vi "OAT Find Time Indices.vi"(7 "reset? (True)":bool=TRUE, 9 "time range":cluster{"start":dbl, "end":dbl, "step":dbl} {"step" format="%.2f"; "end" format="%.2f"; "start" format="%.2f"}, 10 "pulse/revolution (1)":i32=1, 11 "speed profile":T1 {"speed [RPM]" format="%.2f"; "time [s]" format="%.2f"}) -> (0 "finished":bool, 1 "time scale":cluster{"offset":dbl, "multiplier":dbl} {"multiplier" format="%.2f"; "offset" format="%.2f"}, 3 "rev indices":dbl[](array[numeric]) format="%.2f", 5 "last revolution":dbl format="%.2f")   [LabVIEW 2017]
uses:
  <vilib>/addons/Sound and Vibration/Order Analysis/Tach Process/SubVIs/speed profile.ctl
  <vilib>/addons/Sound and Vibration/Order Analysis/Tach Process/SoundVib_TachProcess.lvlib
panel:
  out "missing":bool
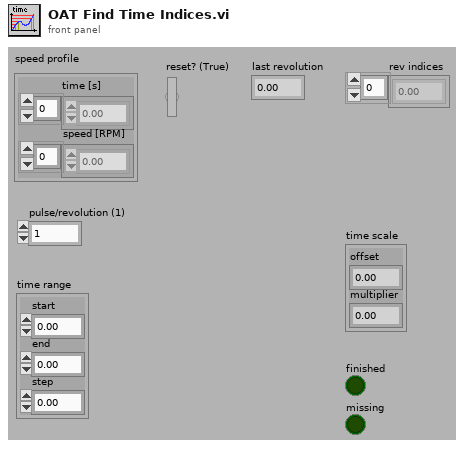
[diagram p1: front panel]
types:
  T1 = typedef "SoundVib_TachProcess.lvlib/speed profile.ctl" = cluster{"time [s]":dbl[], "speed [RPM]":dbl[]}
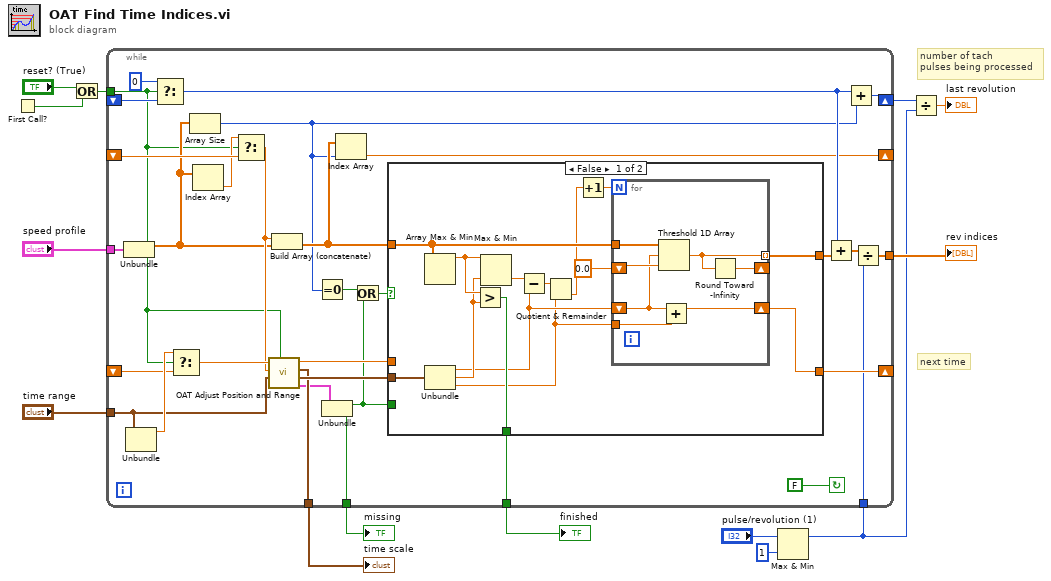
[diagram p0: block diagram]
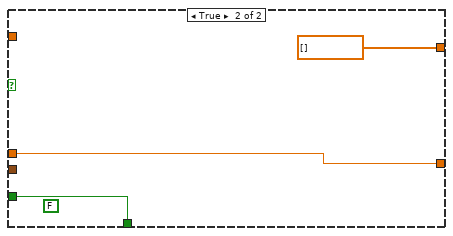
[diagram p2: hidden frame]
diagram:
  # "next time"
  # "number of tach\npulses being processed"
  n1 = First Call?() -> (First Call?: T/F=w10:bool)
  n2 = Or(x="reset? (True)", y=w10) -> (x .or. y?=w11:bool)
  n3 = Max & Min(x="pulse/revolution (1)", y=1) -> (max(x,y)=w4:i32)  [unwired: 1 out]
  n4 = while {
    tunnel: "speed profile" -> [w46]
    tunnel: "time range" -> [w34]
    tunnel: [w42] -> w9
    tunnel: w11 -> [w15]
    shift-right: [w40] -> w7
    shift-left: _ -> [w41]
    shift-right: [w24] -> _
    shift-left: _ -> [w37]
    tunnel: [w31] -> w8
    shift-right: [w25] -> _
    shift-left: _ -> [w29]
    tunnel: w4 -> [w23]
    tunnel: [w18] -> w2
    tunnel: [w17] -> w1
    stop <- FALSE continue-if-true
    n5 = Unbundle(w46) -> ("time [s]"=w16:dbl[])  [unwired: 1 out]
    n6 = Unbundle(w34) -> ("start"=w38:dbl)  [unwired: 2 out]
    n7 = Select(t=0, s=w15, f=w41) -> (s? t:f=w39:i32)
    n8 = Select(t=w38, s=w15, f=w37) -> (s? t:f=w35:dbl)
    n9 = Array Size(array=w16) -> (size(s)=w22:i32)
    n10 = Index Array(array=w16) -> (element=w28:dbl)  [unwired: 1 in]
    n11 = Select(t=w28, s=w15, f=w29) -> (s? t:f=w26:dbl)
    n12 = call <vilib>:"OAT Adjust Position and Range.vi"("reset"=w15, "range in"=w34, "start position"=w26, "current position"=w35) -> ("flags"=w30:cluster{"finished":bool, "data missed":bool}, "range out"=w33:cluster{"start":dbl, "end":dbl, "step":dbl}, "scale"=w31:cluster{"offset":dbl, "multiplier":dbl}, "current position out"=w32:dbl)  [unwired: 4 in]
    n13 = Build Array (concatenate)(w26, w16) -> (w27:dbl[])
    n14 = Equal To 0?(x=w22) -> (x = 0?=w21:bool)
    n15 = Unbundle(w30) -> ("finished"=w19:bool, "data missed"=w18:bool)
    n16 = Index Array(array=w27, index=w22) -> (element=w25:dbl)
    n17 = Or(x=w21, y=w19) -> (x .or. y?=w20:bool)
    n18 = case shown="False" w20 {
      tunnel: w33 -> [w60 _]
      tunnel: w27 -> [w58 _]
      tunnel: [w47 w69] -> w24
      tunnel: [w48 dbl[] []] -> w44
      tunnel: [w55 w68] -> w17
      tunnel: w32 -> [_ w69]
      tunnel: w19 -> [_ w68]
      frame False {
        n19 = Array Max & Min(array=w58) -> (max value=w57:dbl)  [unwired: 3 out]
        n20 = Unbundle(w60) -> ("start"=w53:dbl, "end"=w56:dbl, "step"=w51:dbl)
        n21 = Greater?(x=w57, y=w56) -> (0:w55:bool)
        n22 = Max & Min(x=w57, y=w56) -> (min(x,y)=w54:dbl)  [unwired: 1 out]
        n23 = Subtract(x=w54, y=w53) -> (x-y=w52:dbl)
        n24 = Quotient & Remainder(x=w52, y=w51) -> (floor(x/y)=w50:dbl)  [unwired: 1 out]
        n25 = Increment(x=w50) -> (x+1=w49:dbl)
        n26 = for {
          N: w49 -> [_]
          tunnel: w58 -> [w67]
          shift-right: [w64] -> w47
          shift-left: w53 -> [w63]
          shift-right: [w62] -> _
          shift-left: 0.0 -> [w66]
          tunnel: w51 -> [w65]
          tunnel: [w61] -> w48 mode=indexing
          n27 = Threshold 1D Array(1:w66, 2:w63, 3:w67) -> (0:w61:dbl)
          n28 = Add(x=w63, y=w65) -> (x+y=w64:dbl)
          n29 = Round Toward -Infinity(1:w61) -> (0:w62:dbl)
        }
      }
      frame True {
        (unwired) FALSE
      }
    }
    n30 = Add(x=w39, y=w44) -> (x+y=w43:dbl[])
    n31 = Add(x=w39, y=w22) -> (x+y=w40:i32)
    n32 = Divide(x=w43, y=w23) -> (x/y=w42:dbl[])
  }
  "rev indices" <- w9
  "time scale" <- w8
  "missing" <- w2
  "finished" <- w1
  n33 = Divide(x=w7, y=w4) -> (x/y=→"last revolution":dbl)
